vi "IncludeProject_WhitelistContainsFile.vi"(10 "expected_file":path) -> (0 "error out":errorcluster)   [LabVIEW 2017, in "WhitelistTest.lvlib"]
uses:
  WhitelistTest.lvlib
  Whitelist/Whitelist.lvclass
  Assertion/Assertion.lvlib
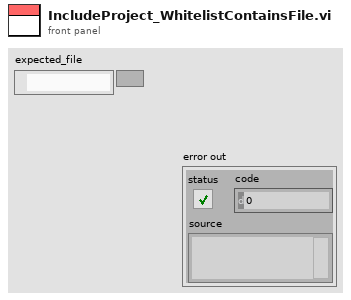
[diagram p1: front panel]
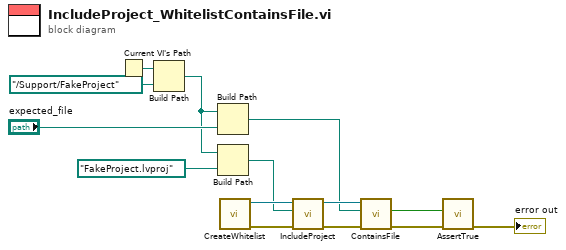
[diagram p0: block diagram]
diagram:
  n1 = Current VI's Path() -> (path=w6:path)
  n2 = Build Path(base path=w6, name or relative path=path "../Support/FakeProject" ("base path")) -> (appended path=w4:path)
  n3 = Build Path(base path=w4, name or relative path="expected_file") -> (appended path=w1:path)
  n4 = Build Path(base path=w4, name or relative path=path "FakeProject.lvproj") -> (appended path=w2:path)
  n5 = call "CreateWhitelist.vi"() -> ("error out"=w11:errorcluster, "Whitelist out"=w9:refnum<class "Whitelist.lvclass">)  [unwired: 10 in]
  n6 = call "IncludeProject.vi"("error in (no error)"=w11, "Path"=w2, "Whitelist in"=w9) -> ("error out"=w10:errorcluster, "Whitelist out"=w8:refnum<class "Whitelist.lvclass">)  [unwired: 7 in]
  n7 = call "ContainsFile.vi"("error in (no error)"=w10, "Path"=w1, "Whitelist in"=w8) -> ("error out"=w14:errorcluster, "Is Whitelisted?"=w13:bool)  [unwired: 6 in, 1 out]
  n8 = call "AssertTrue.vi"("error in (no error)"=w14, "Condition"=w13) -> ("error out"=→"error out":errorcluster)  [unwired: 9 in]
